vi "Write Temperature Status.vi"(8 "error in (no error)":errorcluster, 10 "Temperature Status":T1, 11 "Interface in":refnum<class "Interface.lvclass">) -> (0 "error out":errorcluster, 3 "Interface out":refnum<class "Interface.lvclass">)   [LabVIEW 2018, in "Interface.lvclass"]
uses:
  Interface.lvclass
  Interface.lvclass/Interface.ctl
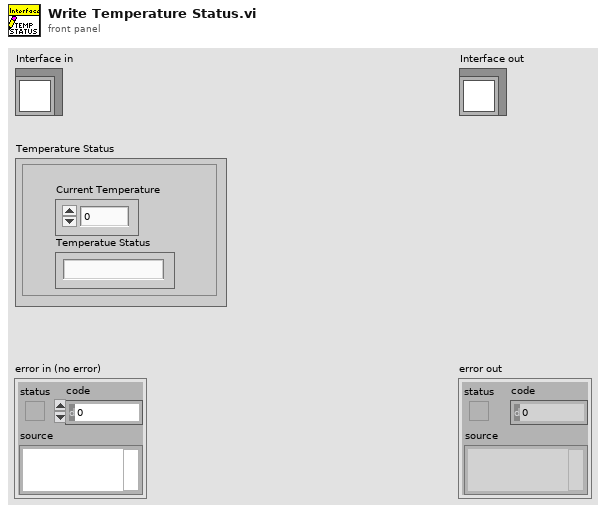
[diagram p1: front panel]
types:
  T1 = cluster{"Current Temperature":i16, "Temperatue Status":string}
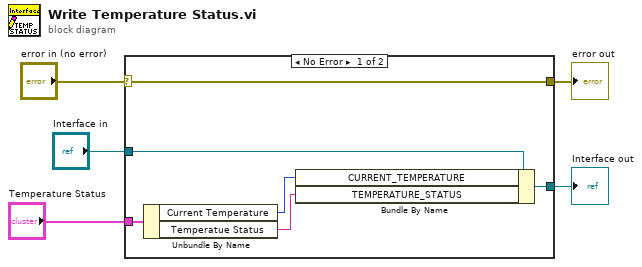
[diagram p0: block diagram]
diagram:
  n1 = case shown="No Error" "error in (no error)" {
    selector: "error in (no error)" -> [w11 w12]
    tunnel: [w11 w12] -> w4
    tunnel: [w9 w13] -> w2
    tunnel: "Interface in" -> [w10 w13]
    tunnel: "Temperature Status" -> [w8 _]
    frame No Error {
      n2 = Unbundle By Name(w8) -> ("Current Temperature"=w6:i16, "Temperatue Status"=w7:string)
      n3 = Bundle By Name(cluster=w10, "CURRENT_TEMPERATURE"=w6, "TEMPERATURE_STATUS"=w7) -> (w9:refnum<class "Interface.lvclass">)
    }
    frame Error {
    }
  }
  "error out" <- w4
  "Interface out" <- w2
